vi "decimateROIs.vi"(11 "ROI_Information_Cluster":T1 {"Norm. XYZ Coordinates"."Apparent Frame Size" format="%#_6f"; "Norm. XYZ Coordinates"."Original FOV (um)" format="%#_6f"; "Norm. XYZ Coordinates"."Pixels per miniscan" format="%#_6f"; "Norm. XYZ Coordinates"."Dwell Time per pixel" format="%#_6f"; "Norm. XYZ Coordinates"."Resolution" format="%#_6f"; "Norm. XYZ Coordinates"."ROI group ID" format="%#_6f"; "Norm. XYZ Coordinates"."Laser Power (%)" format="%#_6f"; "Norm. XYZ Coordinates"."Zoom" format="%#_6f"; "Norm. XYZ Coordinates"."Frame Size" format="%#_6f"; "Norm. XYZ Coordinates"."Number of lines" format="%#_6f"; "Norm. XYZ Coordinates"."Composite ID" format="%#_6f"; "XYZ Coordinates"."Apparent Frame Size" format="%#_6f"; "XYZ Coordinates"."Original FOV (um)" format="%#_6f"; "XYZ Coordinates"."Pixels per miniscan" format="%#_6f"; "XYZ Coordinates"."Dwell Time per pixel" format="%#_6f"; "XYZ Coordinates"."Resolution" format="%#_6f"; "XYZ Coordinates"."ROI group ID" format="%#_6f"; "XYZ Coordinates"."Laser Power (%)" format="%#_6f"; "XYZ Coordinates"."Zoom" format="%#_6f"; "XYZ Coordinates"."Frame Size" format="%#_6f"; "XYZ Coordinates"."Number of lines" format="%#_6f"; "XYZ Coordinates"."Composite ID" format="%#_6f"}) -> (0 "miniScanXYZ":dbl[][](array[numeric]), 1 "miniScan":dbl[](array[numeric]), 2 "POI XYZ":dbl[][](array[numeric]), 3 "POI":dbl[](array[numeric]))   [LabVIEW 2020]
uses:
  Typedefs/Controls/ROI_Information.ctl
  Visualisation/Functional Imaging Viewer/Typedefs/ROI parameters data type.ctl
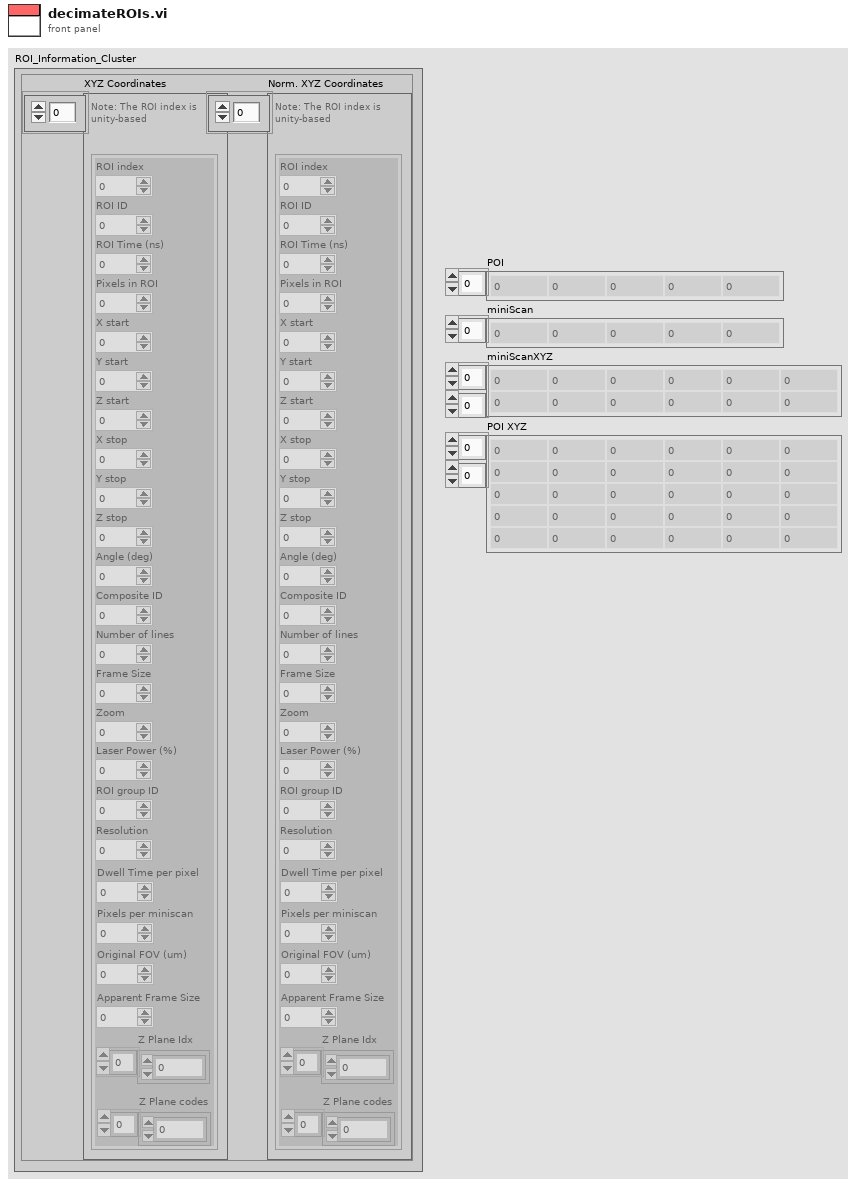
[diagram p1: front panel]
types:
  T1 = typedef "ROI_Information.ctl" = cluster{"XYZ Coordinates":T2[], "Norm. XYZ Coordinates":T2[]}
  T2 = typedef "ROI parameters data type.ctl" = cluster{"ROI index":dbl, "ROI ID":dbl, "ROI Time (ns)":dbl, "Pixels in ROI":dbl, "X start":dbl, "Y start":dbl, "Z start":dbl, "X stop":dbl, "Y stop":dbl, "Z stop":dbl, "Angle (deg)":dbl, "Composite ID":dbl, "Number of lines":dbl, "Frame Size":dbl, "Zoom":dbl, "Laser Power (%)":dbl, "ROI group ID":dbl, "Resolution":dbl, "Dwell Time per pixel":dbl, "Pixels per miniscan":dbl, "Original FOV (um)":dbl, "Apparent Frame Size":dbl, "Z Plane Idx":i32[], "Z Plane codes":i32[]}
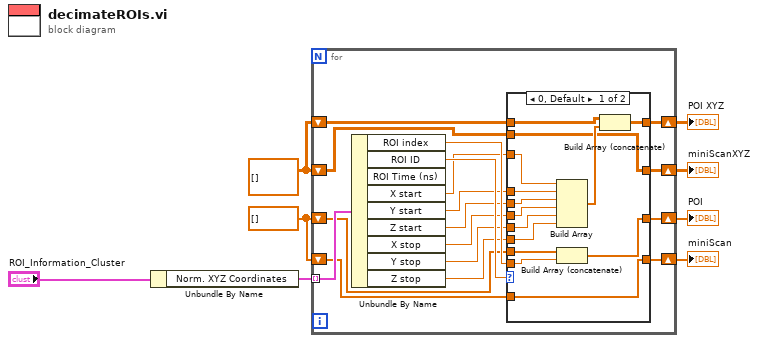
[diagram p0: block diagram]
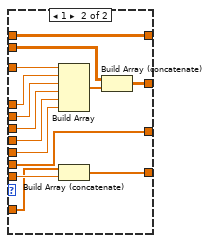
[diagram p2: hidden frame]
diagram:
  w3 = dbl[][] []
  w6 = dbl[] []
  n1 = Unbundle By Name("ROI_Information_Cluster") -> ("Norm. XYZ Coordinates"=w7:T2[])
  n2 = for {
    tunnel: w7 -> [w25] mode=indexing
    shift-right: [w22] -> w5
    shift-left: w6 -> [w21]
    shift-right: [w20] -> w4
    shift-left: w6 -> [w19]
    shift-right: [w12] -> w2
    shift-left: w3 -> [w11]
    shift-right: [w10] -> w1
    shift-left: w3 -> [w9]
    n3 = Unbundle By Name(w25) -> ("ROI index"=w23:dbl, "ROI ID"=w24:dbl, "X start"=w18:dbl, "Y start"=w17:dbl, "Z start"=w16:dbl, "X stop"=w15:dbl, "Y stop"=w14:dbl, "Z stop"=w13:dbl)  [unwired: 1 out]
    n4 = case shown="0, Default" w24 {
      tunnel: w23 -> [w39 w52]
      tunnel: [w38 w53] -> w22
      tunnel: w21 -> [w37 w53]
      tunnel: [w36 w51] -> w20
      tunnel: w19 -> [w36 w50]
      tunnel: w18 -> [w35 w48]
      tunnel: w17 -> [w34 w47]
      tunnel: w16 -> [w33 w46]
      tunnel: w15 -> [w32 w45]
      tunnel: w14 -> [w31 w44]
      tunnel: w13 -> [w30 w43]
      tunnel: [w28 w49] -> w12
      tunnel: w11 -> [w27 w49]
      tunnel: [w26 w41] -> w10
      tunnel: w9 -> [w26 w40]
      frame 0, Default {
        n5 = Build Array(w35, w34, w33, w32, w31, w30) -> (w29:dbl[])
        n6 = Build Array (concatenate)(w37, w39) -> (w38:dbl[])
        n7 = Build Array (concatenate)(w27, w29) -> (w28:dbl[][])
      }
      frame 1 {
        n8 = Build Array(w48, w47, w46, w45, w44, w43) -> (w42:dbl[])
        n9 = Build Array (concatenate)(w50, w52) -> (w51:dbl[])
        n10 = Build Array (concatenate)(w40, w42) -> (w41:dbl[][])
      }
    }
  }
  "POI" <- w5
  "miniScan" <- w4
  "POI XYZ" <- w2
  "miniScanXYZ" <- w1
